vi "Edge Detection - Copy.vi"() -> ()   [LabVIEW 2016]
doc: "This example shows how to use the Edge Tool in NI Vision. The Edge Tool finds edges (or sharp transitions in the pixels values) along a given line or ROI profile. The Edge Tool is a precursor function to many of the gauging and inspection tasks. For example, the location of the edges found along a line profile across an object can interpreted as the boundaries of the object whose dimensions have to be measured for a gauging application or the presence of a crack in the surface of an object for an inspection application."
uses:
  <vilib>/vision/NI_Vision_Development_Module.lvlib
panel:
  in  "Path":path=path "C:/Users/TTUHEP/Documents/LabVIEW/image3.png"
  out "Line Equation":cluster{"A":dbl, "B":dbl, "C":dbl} {"C" format="%.2f"; "B" format="%.2f"; "A" format="%.2f"}
  in  "Process":u16(ring) items=["Get First Edge", "Get First + Last Edge", "Get All Edges", "Get Best Edge"]
  in  "Edge Options":T1={"Edge Polarity"=2, "Kernel Size"=37, "Width"=5, "Minimum Edge Strength"=10.0, "Interpolation Type"=0, "Data Processing Method"=1} {"Data Processing Method" items=["Average", "Median"]; "Interpolation Type" items=["Zero Order"=0, "Bilinear"=1, "Bilinear Fixed"=4]; "Minimum Edge Strength" min=0.0 max=255.0 format="%.2g"; "Width" min=1 step=2; "Kernel Size" min=3 step=2; "Edge Polarity" items=["All Edges", "Rising Edges", "Falling Edges"]}
  out "Image":T2(plugin-control)
  out "Line Profile":cluster{"x0":sgl, "dx":sgl, "Pixels Line":sgl[]}(graph)
  in  "Stop":bool
  # "Overview: Demonstrates how to use the IMAQ Edge Tool function to find edges along a Region of Interest (ROI).\nRequirements: Vision Development Software.\nInstructions:\n1. Run the VI.\n2. Draw a ROI in the image or change the Process or Edge Options to see the edges detected along the ROI."
  # "Ax + By + C = 0"
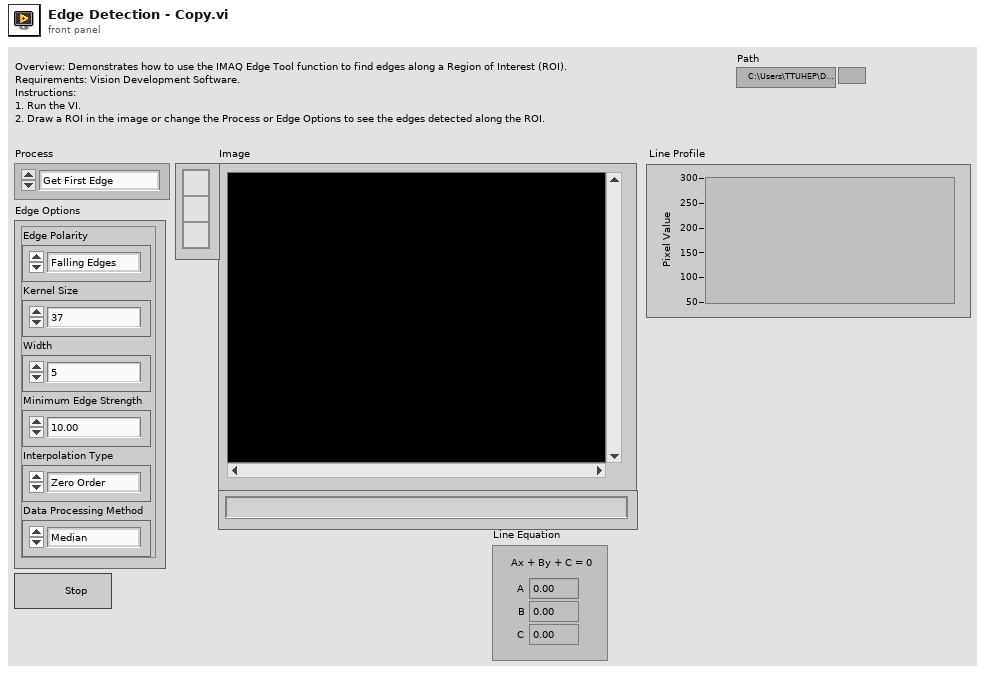
[diagram p1: front panel]
types:
  T1 = cluster{"Edge Polarity":u16, "Kernel Size":u32, "Width":u32, "Minimum Edge Strength":dbl, "Interpolation Type":u16, "Data Processing Method":u16}
  T2 = typedef "IMAQ Image.ctl" = refnum<image>
  T3 = typedef "IMAQ Line" = cluster{"Start X":i32, "Start Y":i32, "End X":i32, "End Y":i32}
  T4 = typedef "ROI Descriptor" = cluster{"Global Rectangle":i32[], "Contours":cluster{"ID":enum32{"External", "Internal"}, "Type":u32, "Coordinates":i32[]}[]}
  T5 = cluster{"Global Rectangle":i32[], "Contours":cluster{"Contour Type":u32, "ROI Type":u32, "Points":i32[]}[]}
  T6 = typedef "Edge New.ctl" = cluster{"Location (Pixel)":cluster{"X":sgl, "Y":sgl}, "Location (Real-World)":cluster{"X":sgl, "Y":sgl}, "Distance (Pixel)":dbl, "Distance (Real-World)":dbl, "Strength":dbl, "Noise":dbl, "Rising?":bool}
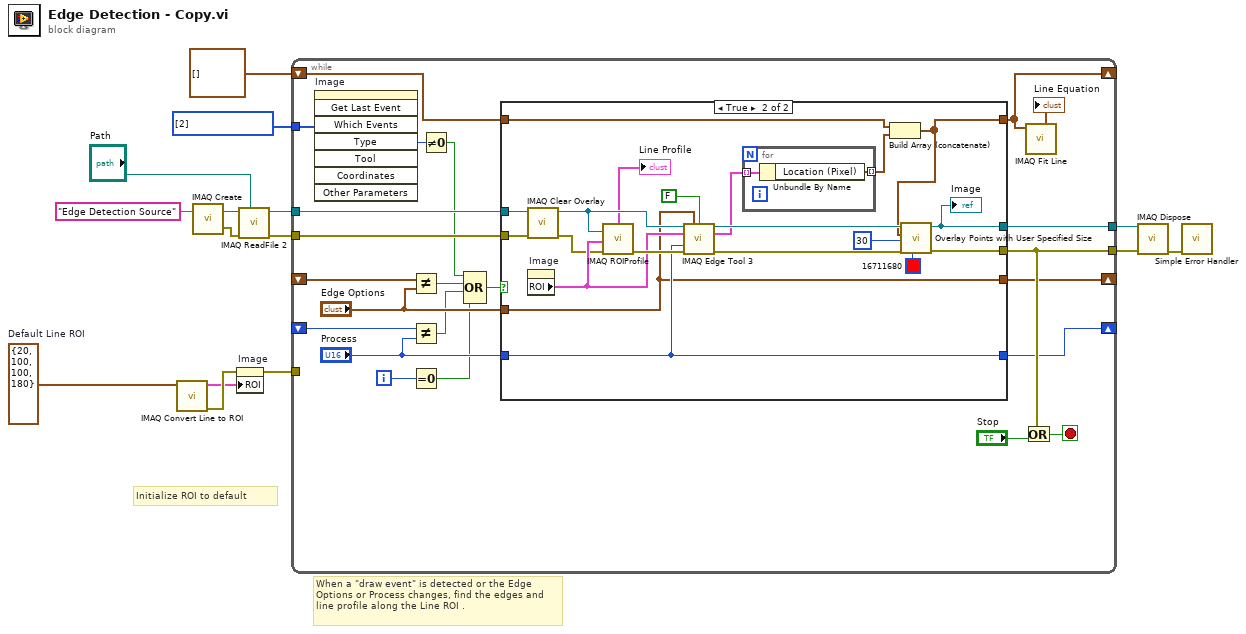
[diagram p0: block diagram]
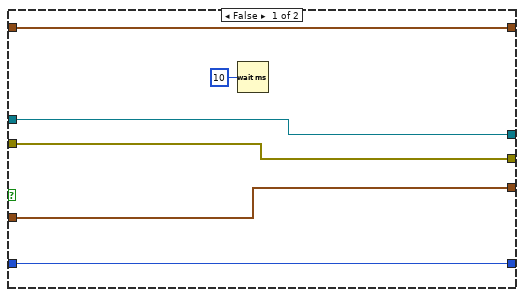
[diagram p2: hidden frame]
diagram:
  w1 = T3 {"Start X"=20, "Start Y"=100, "End X"=100, "End Y"=180}  # Default Line ROI
  w7 = i32[] [2] items=["No  event", "Click event", "Draw event", "Move event", "Size event", "Scroll event", "Activate event", "Close event", "Double click event"] ("Events list (all)")
  # "Initialize ROI to default"
  # "When a \"draw event\" is detected or the Edge Options or Process changes, find the edges and line profile along the Line ROI ."
  n1 = call "IMAQ Convert Line to ROI"("Line"=w1) -> ("error out"=w6:errorcluster, "ROI Descriptor"=w5:T4)  [unwired: 8 in]
  n2 = call "IMAQ Create"("Image Name"="Edge Detection Source") -> ("New Image"=w14:T2, "error out"=w13:errorcluster)  [unwired: 4 in]
  n3 = property on="Image" class="ImageControl"(error in=w6, "ROI"=w5) -> (error out=w4:errorcluster)  [unwired: 1 in, 1 out]
  n4 = call "IMAQ ReadFile 2"("File Path"="Path", "error in (no error)"=w13, "Image"=w14) -> ("error out"=w8:errorcluster, "Image Out"=w9:T2)  [unwired: 4 in, 3 out]
  n5 = while {
    tunnel: w9 -> [w37]
    tunnel: w8 -> [w38]
    tunnel: [w33] -> w12
    tunnel: [w34] -> w11
    tunnel: w7 -> [w32]
    shift-right: [w19] -> _
    shift-left: _ -> [w29]
    shift-right: [w20] -> _
    shift-left: _ -> [w27]
    tunnel: w4 -> [_]
    shift-right: [w17] -> _
    shift-left: cluster{"X":sgl, "Y":sgl}[] [] -> [w18]
    i -> [w30]
    stop <- w35 stop-if-true
    n6 = invoke on="Image" class="ImageControl" method="Get Last Event"("Which Events"=w32) -> ("Type"=w31:i32)  [unwired: 7 in, 7 out]
    n7 = Not Equal?(x=w29, y="Edge Options") -> (x != y?=w25:bool)
    n8 = Not Equal?(x=w27, y="Process") -> (x != y?=w24:bool)
    n9 = Equal To 0?(x=w30) -> (x = 0?=w23:bool)
    n10 = Not Equal To 0?(x=w31) -> (x != 0?=w22:bool)
    n11 = Compound Arithmetic op=OR(w22, w25, w24, w23) -> (w21:bool)
    n12 = case shown="True" w21 {
      tunnel: w38 -> [w43 w56]
      tunnel: w37 -> [w44 w55]
      tunnel: [w44 w58] -> w34
      tunnel: [w43 w62] -> w33
      tunnel: "Edge Options" -> [w41 w49]
      tunnel: "Process" -> [w40 w51]
      tunnel: [w40 w51] -> w20
      tunnel: [w41 w49] -> w19
      tunnel: w18 -> [w39 w48]
      tunnel: [w39 w46] -> w17
      frame False {
        n13 = Wait (ms)(milliseconds to wait=u32 10) -> ()  [unwired: 1 out]
      }
      frame True {
        n14 = call "IMAQ Clear Overlay"("error in (no error)"=w56, "Image"=w55) -> ("error out"=w53:errorcluster, "Image Out"=w54:T2)  [unwired: 8 in]
        n15 = property on="Image" class="ImageControl"() -> ("ROI"=w57:T5)  [unwired: 2 in, 2 out]
        n16 = call "IMAQ ROIProfile"("error in (no error)"=w53, "ROI Descriptor"=w57, "Image"=w54) -> ("error out"=w64:errorcluster, "ROI Graph"=→"Line Profile":cluster{"x0":sgl, "dx":sgl, "Pixels Line":sgl[]})  [unwired: 1 in, 3 out]
        n17 = call "IMAQ Edge Tool 3"("Image"=w54, "Edge Options"=w49, "Optimized Mode"=FALSE, "ROI Descriptor"=w57, "Process"=w51, "error in (no error)"=w64) -> ("Image (duplicate)"=w61:T2, "Edge Information"=w60:T6[], "error out"=w63:errorcluster)  [unwired: 5 in, 2 out]
        n18 = for {
          tunnel: w60 -> [w66] mode=indexing
          tunnel: [w65] -> w47 mode=indexing
          n19 = Unbundle By Name(w66) -> ("Location (Pixel)"=w65:cluster{"X":sgl, "Y":sgl})
        }
        n20 = Build Array (concatenate)(w48, w47) -> (w46:cluster{"X":sgl, "Y":sgl}[])
        n21 = call "Overlay Points with User Specified Size.vi"("Color"=u32 16711680, "error in"=w63, "Point Diameter (5)"=30, "Points"=w46, "Image In"=w61) -> ("error out"=w62:errorcluster, "Image Out"=w58:T2)  [unwired: 5 in]
        "Image" <- w58
      }
    }
    n22 = Or(x=w33, y="Stop") -> (x .or. y?=w35:bool)
    n23 = call "IMAQ Fit Line"("Points"=w17) -> ("Line Equation"=→"Line Equation":cluster{"A":dbl, "B":dbl, "C":dbl})  [unwired: 5 in, 5 out]
  }
  n24 = call "IMAQ Dispose"("Image"=w11, "error in (no error)"=w12) -> ("error out"=w10:errorcluster)  [unwired: 4 in]
  n25 = call <vilib>:"Simple Error Handler.vi"("error in (no error)"=w10) -> ()  [unwired: 4 in, 5 out]
